vi "CleanHistory.vi"(11 "History Array In":path[](array[path])) -> (3 "History Array out":path[](array[path]))   [LabVIEW 2009, in "HistoryPath.xctl"]
uses:
  HistoryPath.xctl
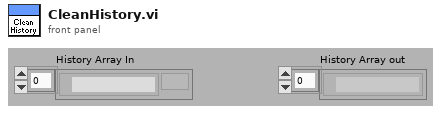
[diagram p1: front panel]
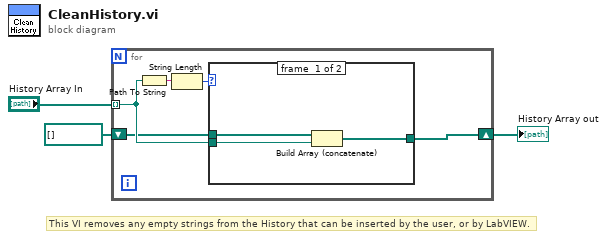
[diagram p0: block diagram]
diagram:
  # "This VI removes any empty strings from the History that can be inserted by the user, or by LabVIEW."
  n1 = for {
    tunnel: "History Array In" -> [w6] mode=indexing
    shift-right: [w5] -> w2
    shift-left: path[] [] -> [w4]
    n2 = Path To String(path=w6) -> (string=w8:string)
    n3 = String Length(string=w8) -> (length=w7:i32)
    n4 = case shown="1, Default" w7 {
      tunnel: w6 -> [w11 _]
      tunnel: [w10 w12] -> w5
      tunnel: w4 -> [w9 w12]
      frame #0 {
        n5 = Build Array (concatenate)(w9, w11) -> (w10:path[])
      }
      frame #1 {
      }
    }
  }
  "History Array out" <- w2
